vi "go_around_right.vi"(8 "error in (no error)":errorcluster) -> (0 "error out 2":errorcluster)   [LabVIEW 2014]
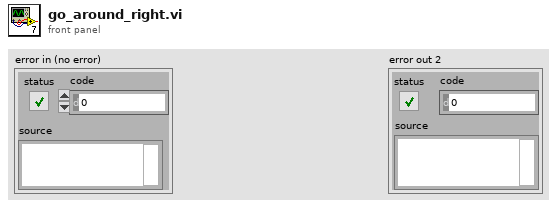
[diagram p1: front panel]
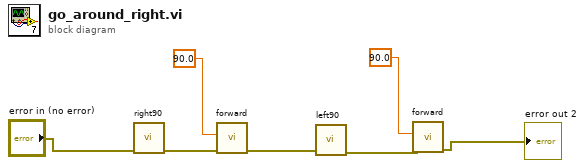
[diagram p0: block diagram]
diagram:
  n1 = call "right90.vi"("error in (no error)"="error in (no error)") -> ("error out"=w6:errorcluster)  [unwired: 10 in]
  n2 = call "forward.vi"("error in (no error)"=w6, "Dist (cm)"=90.0) -> ("error out"=w5:errorcluster)  [unwired: 9 in]
  n3 = call "left90.vi"("error in (no error)"=w5) -> ("error out"=w2:errorcluster)  [unwired: 9 in, 1 out]
  n4 = call "forward.vi"("error in (no error)"=w2, "Dist (cm)"=90.0) -> ("error out"=→"error out 2":errorcluster)  [unwired: 9 in]
